vi "10min.vi"() -> ()   [LabVIEW 2017, in "Examples.lvlib"]
uses:
  Examples.lvlib
  <vilib>/Utility/Variable/NI_VariableUtilities.lvlib
panel:
  out "Logging? 2":bool
  in  "Stop Time":timestamp
  in  "Start Time":timestamp
  out "Waveform Voltage F403013 3":sgl(graph)
  out "Waveform Voltage F403013 2":sgl(graph)
  in  "Stop Button 3":bool
  out "Numeric Indicator 2":dbl
  out "Numeric Indicator":dbl
  out "F403147 2":sgl(graph)
  out "Waveform Voltage F403151":sgl(graph)
  out "Waveform Voltage F403149":sgl(graph)
  out "F403147":sgl(graph)
  in  "Stop Button 2":bool
  out "Iteration":i32
  out "Logging?":bool
  out "Waveform Voltage F403007 2":sgl(graph)
  in  "Stop Button":bool
  out "Waveform Voltage F403007":sgl(graph)
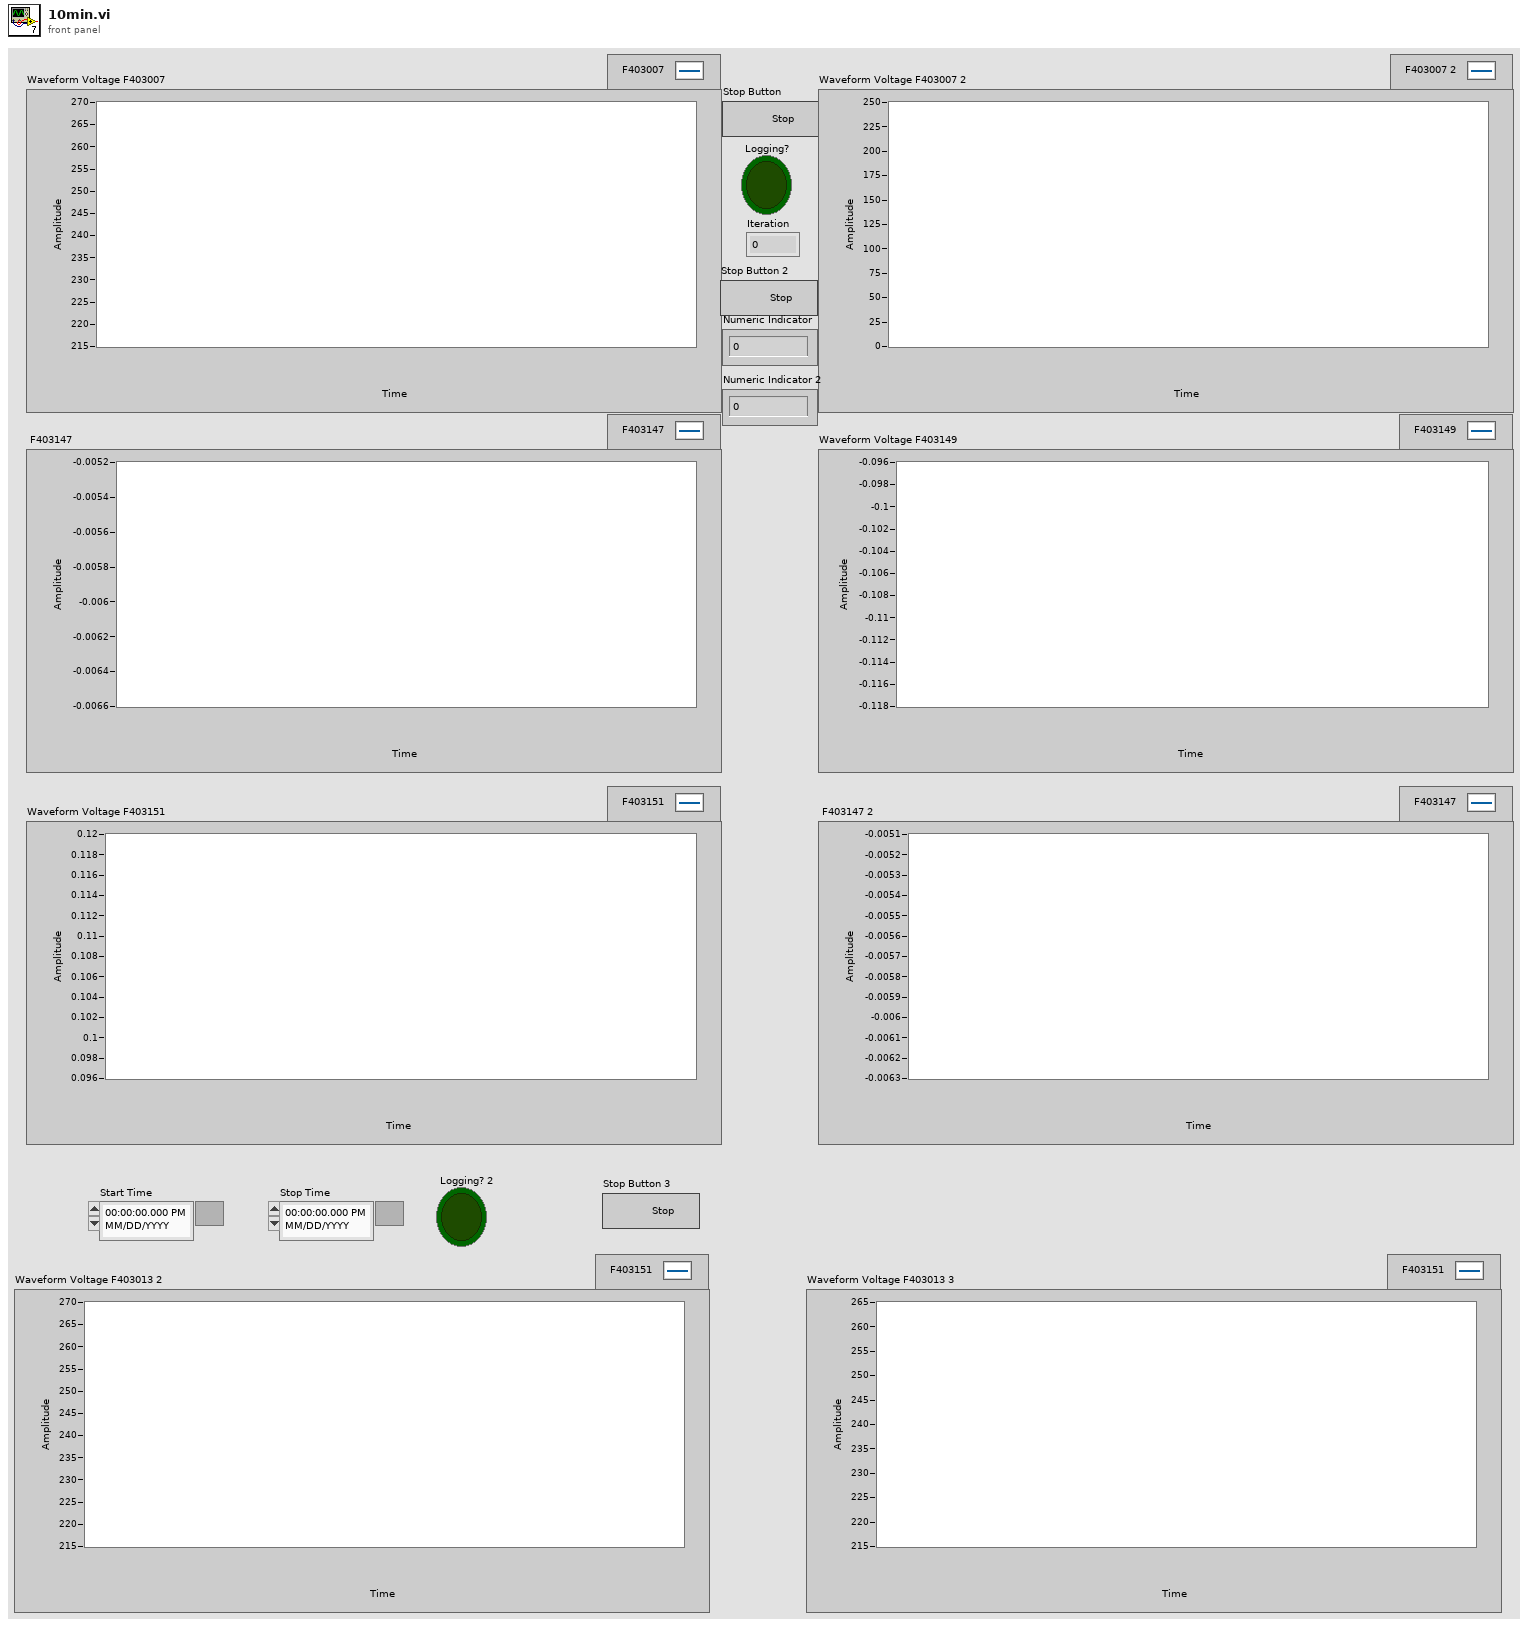
[diagram p1: front panel]
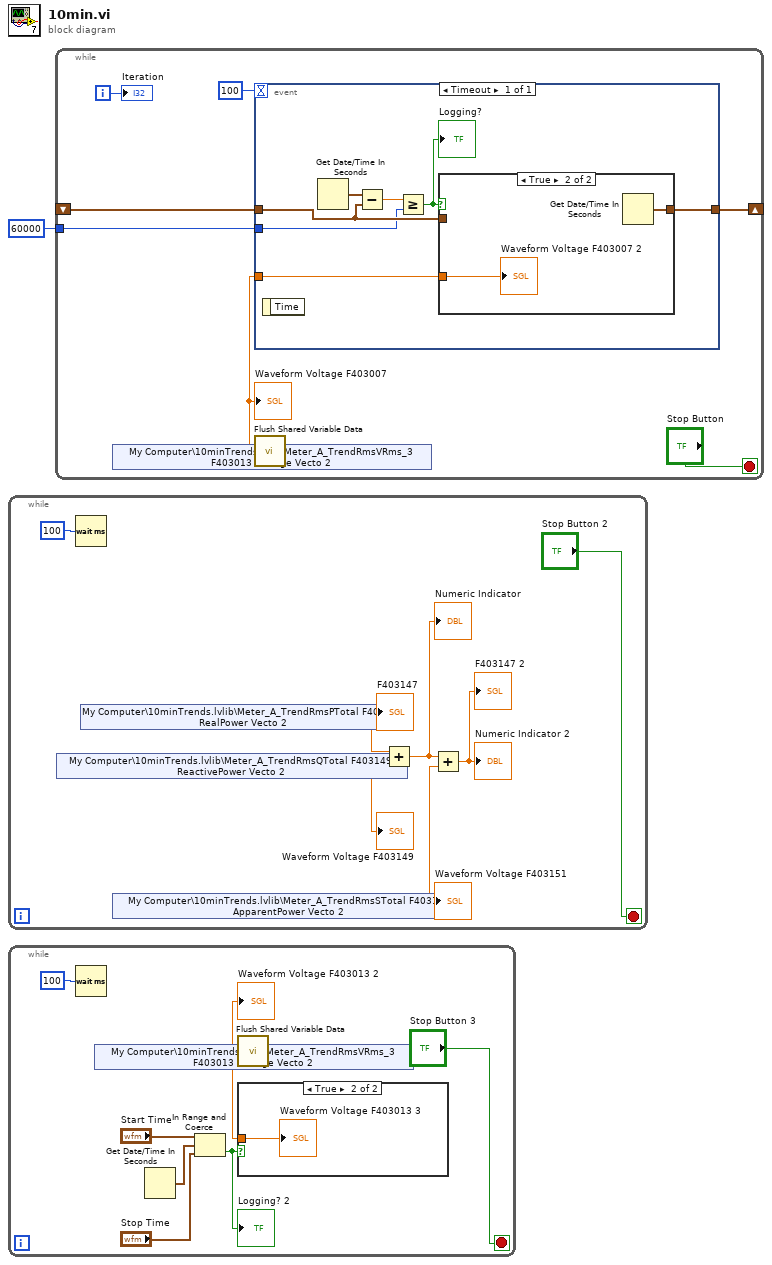
[diagram p0: block diagram]
diagram:
  n1 = while {
    stop <- "Stop Button 2" stop-if-true
    n2 = shared-variable "My Computer\\10minTrends.lvlib\\Meter_A_TrendRmsQTotal F403149 ReactivePower Vecto 2"() -> (w5:sgl)  [unwired: 1 in, 1 out]
    "Waveform Voltage F403149" <- w5
    n3 = Wait (ms)(milliseconds to wait=u32 100) -> ()  [unwired: 1 out]
    n4 = shared-variable "My Computer\\10minTrends.lvlib\\Meter_A_TrendRmsPTotal F403147 RealPower Vecto 2"() -> (w6:sgl)  [unwired: 1 in, 1 out]
    "F403147" <- w6
    n5 = shared-variable "My Computer\\10minTrends.lvlib\\Meter_A_TrendRmsSTotal F403151 ApparentPower Vecto 2"() -> (w4:sgl)  [unwired: 1 in, 1 out]
    "Waveform Voltage F403151" <- w4
    n6 = Add(x=w6, y=w5) -> (x+y=w3:sgl)
    "Numeric Indicator" <- w3
    n7 = Add(x=w3, y=w4) -> (x+y=→"F403147 2" →"Numeric Indicator 2":sgl)
  }
  n8 = while {
    stop <- "Stop Button 3" stop-if-true
    n9 = Wait (ms)(milliseconds to wait=u32 100) -> ()  [unwired: 1 out]
    n10 = shared-variable "My Computer\\10minTrends.lvlib\\Meter_A_TrendRmsVRms_3 F403013 Voltage Vecto 2"() -> (w15:sgl, error out=w9:errorcluster)  [unwired: 1 in]
    "Waveform Voltage F403013 2" <- w15
    n11 = Get Date/Time In Seconds() -> (seconds since 1Jan1904=w14:timestamp)
    n12 = In Range and Coerce(upper limit="Start Time", x=w14, lower limit="Stop Time") -> (In Range?=w11:bool)  [unwired: 1 out]
    "Logging? 2" <- w11
    n13 = call <vilib>:"Flush Shared Variable Data.vi"("error in (no error)"=w9) -> ()  [unwired: 10 in, 1 out]
    n14 = case shown="True" w11 {
      tunnel: w15 -> [_ w17]
      frame False {
      }
      frame True {
        "Waveform Voltage F403013 3" <- w17
      }
    }
  }
  n15 = while {
    tunnel: 60000 -> [w23]
    shift-right: [w21] -> _
    shift-left: _ -> [w22]
    i -> [w24]
    stop <- "Stop Button" stop-if-true
    n16 = shared-variable "My Computer\\10minTrends.lvlib\\Meter_A_TrendRmsVRms_3 F403013 Voltage Vecto 2"() -> (w19:sgl, error out=w18:errorcluster)  [unwired: 1 in]
    "Waveform Voltage F403007" <- w19
    n17 = event shown="[0] Timeout" {
      selector: _ -> [_]
      dyn-events: _ -> [_]
      timeout: 100 -> [_]
      tunnel: w22 -> [w31]
      tunnel: w23 -> [w29]
      tunnel: [w27] -> w21
      tunnel: w19 -> [w26]
      event Timeout {
        n18 = event-data() -> ()  [unwired: 1 in, 1 out]
        n19 = Get Date/Time In Seconds() -> (seconds since 1Jan1904=w32:timestamp)
        n20 = Subtract(x=w32, y=w31) -> (x-y=w30:dbl)
        n21 = Greater Or Equal?(x=w30, y=w29) -> (x >= y?=w28:bool)
        "Logging?" <- w28
        n22 = case shown="True" w28 {
          tunnel: w31 -> [w33 _]
          tunnel: [w33 w35] -> w27
          tunnel: w26 -> [_ w34]
          frame False {
          }
          frame True {
            n23 = Get Date/Time In Seconds() -> (seconds since 1Jan1904=w35:timestamp)
            "Waveform Voltage F403007 2" <- w34
          }
        }
      }
    }
    n24 = call <vilib>:"Flush Shared Variable Data.vi"("error in (no error)"=w18) -> ()  [unwired: 10 in, 1 out]
    "Iteration" <- w24
  }
